vi "convertObjectToCluster__ogtk.vi"(0 "LabVIEW Object in":refnum<class>, 1 "error in (no error)":errorcluster) -> (14 "VCluster":variant, 15 "error out":errorcluster)   [LabVIEW 2023, in "openg_variant.lvlib"]
doc: "Transform object to a flat cluster containing all elements from every class in the hierarchy.\n\nGCraftsman JSON Object Serialization Toolkit\nwww.GCraftsman.com\nCopyright (c) 2017, GCraftsman"
uses:
  openg_variant.lvlib
  Reflection__ogtk.lvclass
panel:
  # "EXPERIMENTAL"
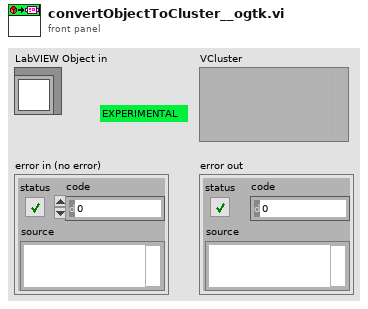
[diagram p1: front panel]
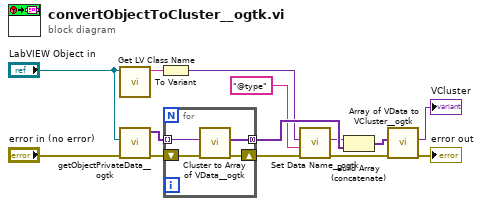
[diagram p0: block diagram]
diagram:
  n1 = call <vilib>:"Get LV Class Name.vi"("object"="LabVIEW Object in") -> ("class name"=w7:string)  [unwired: 9 in, 1 out]
  n2 = call "getObjectPrivateData__ogtk.vi"("error in (no error)"="error in (no error)", "object in"="LabVIEW Object in") -> ("error out"=w11:errorcluster, "privateData"=w14:variant[])  [unwired: 7 in, 1 out]
  n3 = To Variant(anything=w7) -> (Variant=w6:variant)
  n4 = for {
    tunnel: w14 -> [w18] mode=indexing
    tunnel: [w15] -> w8 mode=concatenating
    shift-right: [w16] -> w2
    shift-left: w11 -> [w17]
    n5 = call "Cluster to Array of VData__ogtk.vi"("error in (no error)"=w17, "Cluster"=w18) -> ("error out"=w16:errorcluster, "Array of VData"=w15:variant[])  [unwired: 8 in]
  }
  n6 = call "Set Data Name__ogtk.vi"("error in (no error)"=w2, "Data Name"="@type", "Data"=w6) -> ("error out"=w1:errorcluster, "Renamed Data"=w4:variant)  [unwired: 7 in]
  n7 = Build Array (concatenate)(w4, w8) -> (w3:variant[])
  n8 = call "Array of VData to VCluster__ogtk.vi"("error in (no error)"=w1, "Array"=w3) -> ("error out"=→"error out":errorcluster, "VCluster"=→"VCluster":variant)  [unwired: 8 in]
